vi "Square to string.vi"(11 "Square":T1={"File"=enum."d", "Rank"=enum."4"}) -> (3 "Square string":string)   [LabVIEW 2016, in "Chesslib.lvlib"]
uses:
  Chesslib.lvlib
  typedef/Square.ctl
  typedef/File.ctl
  typedef/Rank.ctl
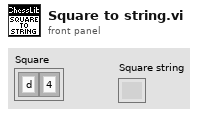
[diagram p1: front panel]
types:
  T1 = typedef "Chesslib.lvlib/Square.ctl" = cluster{"File":T2, "Rank":T3}
  T2 = typedef "Chesslib.lvlib/File.ctl" = enum8{"a", "b", "c", "d", "e", "f", "g", "h"}
  T3 = typedef "Chesslib.lvlib/Rank.ctl" = enum8{"1", "2", "3", "4", "5", "6", "7", "8"}
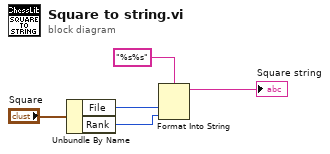
[diagram p0: block diagram]
diagram:
  n1 = Unbundle By Name("Square") -> ("File"=w4:T2, "Rank"=w3:T3)
  n2 = Format Into String(format string="%s%s", w4, w3) -> (resulting string=→"Square string":string)  [unwired: 2 in, 1 out]
